vi "RM.searchServerInfoArrayByGUID.vi"(8 "error in (no error)":errorcluster, 10 "selected deviceGUID":string, 11 "serverInfo array in":T1[](array[typedef]) {"cd node ref" format="%.0x"}) -> (0 "error out":errorcluster, 1 "found?":bool, 2 "serverInfo":T1 {"cd node ref" format="%.0x"}, 3 "serverInfo array out":T1[](array[typedef]) {"cd node ref" format="%.0x"})   [LabVIEW 2016, in "FPGA Resource Manager.lvlib"]
uses:
  FPGA Resource Manager.lvlib
  RM.serverInfo.ctl
  <vilib>/NI Veristand/Custom Device API/Custom Device Item Ref.ctl
  <vilib>/NI Veristand/Custom Device API/Custom Device API.lvlib
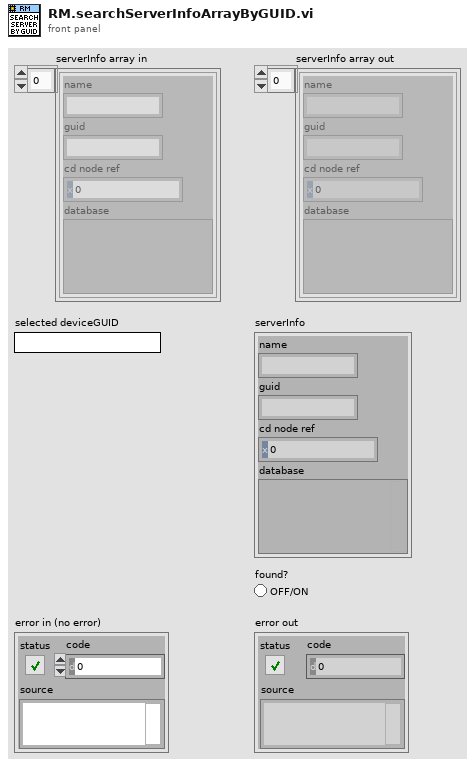
[diagram p1: front panel]
types:
  T1 = typedef "FPGA Resource Manager.lvlib/RM.serverInfo.ctl" = cluster{"name":string, "guid":string, "cd node ref":T2, "database":variant}
  T2 = typedef "Custom Device API.lvlib/Custom Device Item Ref.ctl" = u64
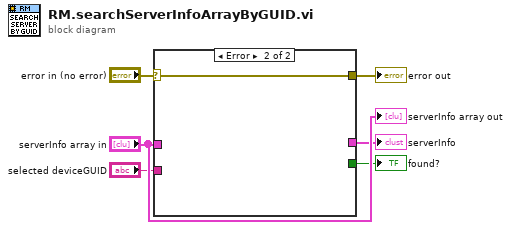
[diagram p0: block diagram]
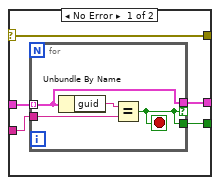
[diagram p2: hidden frame]
diagram:
  n1 = case shown="Error" "error in (no error)" {
    selector: "error in (no error)" -> [w7 w16]
    tunnel: "serverInfo array in" -> [w11 _]
    tunnel: "selected deviceGUID" -> [w10 _]
    tunnel: [w9 _] -> w4
    tunnel: [w8 _] -> w3
    tunnel: [w7 w16] -> w1
    frame No Error {
      n2 = for {
        tunnel: w11 -> [w12] mode=indexing
        tunnel: w10 -> [w14]
        tunnel: [w12] -> w8 if=w13
        tunnel: [w13] -> w9
        stop <- w13 stop-if-true
        n3 = Unbundle By Name(w12) -> ("guid"=w15:string)
        n4 = Equal?(x=w15, y=w14) -> (x = y?=w13:bool)
      }
    }
    frame Error {
    }
  }
  "found?" <- w4
  "serverInfo" <- w3
  "error out" <- w1
  "serverInfo array out" <- "serverInfo array in"
